vi "OAT Easy Significant Gabor Order Tracking (Digital Tach).vi"(0 "scaled signal [EU]":waveform(dbl)={"t0"=timestamp(0 s since 1904-01-01), "dt"=0.0, "Y"=[]}, 1 "bandwidth":T4={"bandwidth value"=0.5, "bandwidth unit"=enum."Order"} {"bandwidth value" min=0.0 format="%.2f"}, 2 "window info in (auto)":T1={"window type"=10, "window length"=0} {"window type" items=["None"=0, "Hanning"=1, "Hamming"=2, "Blackman-Harris"=3, "Exact Blackman"=4, "Blackman"=5, "Flat Top"=6, "4 Term B-Harris"=7, "7 Term B-Harris"=8, "Low Sidelobe"=9, "Gaussian"=62]; "window length" min=0}, 5 "number of orders (3)":i32=3, 7 "digital tach info":T5={"tacho counts"=[], "counter timebase [Hz]"=20000000.0, "counter task type"=enum."event counting", "counter digit (32)"=32}, 9 "pulse/revolution (1)":i32=1, 11 "error in (no error)":errorcluster, 12 "X axis selection":u16(ring)=2 items=["Time", "Revolution", "RPM"], 13 "phase setting":T2) -> (3 "samples/rev":dbl format="%.2f", 4 "magnitudes (RMS)":cluster{"X":dbl[], "Y":dbl[]}[](array[cluster]) {"Y" format="%.2f"; "X" format="%.2f"}, 6 "phase lags":cluster{"X":dbl[], "Y":dbl[]}[](array[cluster]) {"Y" format="%.2f"; "X" format="%.2f"}, 8 "order waveforms [EU]":waveform(dbl)[](array[waveform]), 10 "unit labels":T3, 14 "orders":dbl[](array[numeric]) format="%.2f", 15 "error out":errorcluster)   [LabVIEW 2017]
doc: "Extracts the most significant orders from <B>scaled signal [EU]</B> and computes <B>magnitudes</B> and <B>phase lags</B> for the significant orders. You can use this polymorphic VI to perform significant order tracking for an analog tachometer signal or a digital tachometer signal. The data type you wire to the <B>analog tach signal</B> input determines the polymorphic instance to use."
uses:
  <vilib>/addons/Sound and Vibration/Order Analysis/Tach Process/SubVIs/digital tach info.ctl
  <vilib>/addons/Sound and Vibration/Order Analysis/Ref Gabor Order Tracking/Mask Bandwidth.ctl
  <vilib>/addons/Sound and Vibration/Order Analysis/Ref Gabor Order Tracking/window information.ctl
  <vilib>/addons/Sound and Vibration/Order Analysis/Tach Process/SubVIs/speed profile.ctl
  <vilib>/addons/Sound and Vibration/Order Analysis/Tach Process/SoundVib_TachProcess.lvlib
  <vilib>/addons/Sound and Vibration/Order Analysis/Gabor Order Tracking/SoundVib_Gabor.lvlib
panel:
  # "OAT Easy Significant Gabor Order Tracking (Digital Tach)"
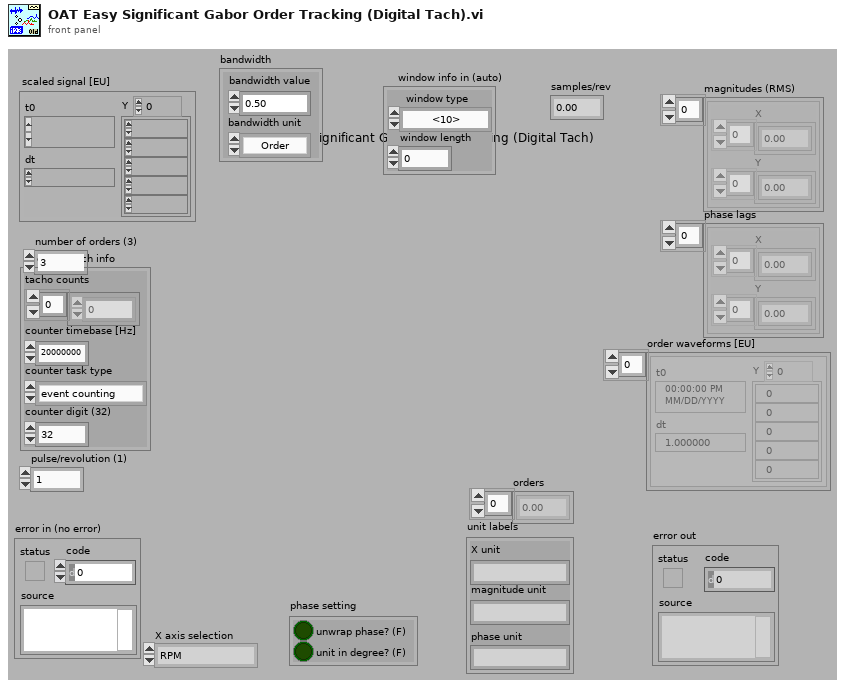
[diagram p1: front panel]
types:
  T1 = typedef "SoundVib_Gabor.lvlib/window information.ctl" = cluster{"window type":u32, "window length":i32}
  T2 = cluster{"unwrap phase? (F)":bool, "unit in degree? (F)":bool}
  T3 = cluster{"X unit":string, "magnitude unit":string, "phase unit":string}
  T4 = typedef "SoundVib_Gabor.lvlib/Mask Bandwidth.ctl" = cluster{"bandwidth value":dbl, "bandwidth unit":enum16{"Order", "Hz"}}
  T5 = typedef "SoundVib_TachProcess.lvlib/digital tach info.ctl" = cluster{"tacho counts":i64[], "counter timebase [Hz]":dbl, "counter task type":enum16{"period measurement", "event counting"}, "counter digit (32)":i32}
  T6 = typedef "SoundVib_TachProcess.lvlib/speed profile.ctl" = cluster{"time [s]":dbl[], "speed [RPM]":dbl[]}
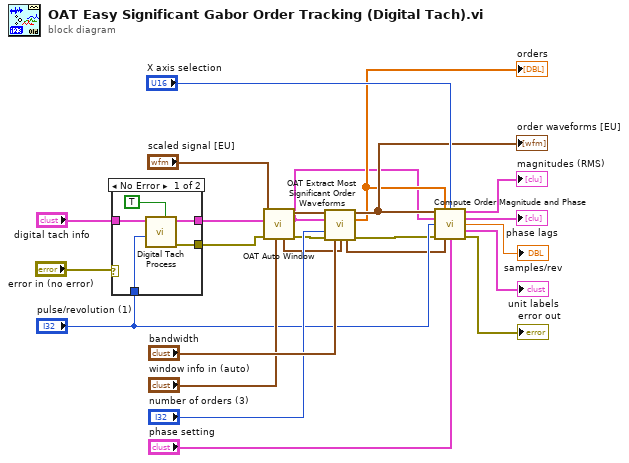
[diagram p0: block diagram]
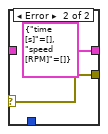
[diagram p2: hidden frame]
diagram:
  n1 = case shown="No Error" "error in (no error)" {
    selector: "error in (no error)" -> [_ w30]
    tunnel: "digital tach info" -> [w29 _]
    tunnel: "pulse/revolution (1)" -> [w28 _]
    tunnel: [w27 T6 {"time [s]"=[], "speed [RPM]"=[]} ("speed profile")] -> w10
    tunnel: [w26 w30] -> w7
    frame No Error {
      n2 = call <vilib>:"Digital Tach Process.vi"("reset? (True)"=TRUE ("reset? (False)"), "pulse/revolution (1)"=w28, "digital tach info"=w29) -> ("error out"=w26:errorcluster, "speed profile"=w27:T6)  [unwired: 6 in, 1 out]
    }
    frame Error {
    }
  }
  n3 = call <vilib>:"OAT Auto Window.vi"("window info in"="window info in (auto)", "error in (no error)"=w7, "speed profile"=w10, "scaled signal [EU]"="scaled signal [EU]") -> ("error out"=w6:errorcluster, "speed profile out"=w3:T6, "scaled signal [EU] out"=w11:waveform(dbl), "window info out"=w9:T1)  [unwired: 4 in]
  n4 = call <vilib>:"OAT Extract Most Significant Order Waveforms.vi"("scaled signal [EU]"=w11, "speed profile"=w3, "number of orders (3)"="number of orders (3)", "error in (no error)"=w6, "bandwidth"="bandwidth", "window info"=w9) -> ("order waveforms [EU]"=w19:waveform(dbl)[], "orders"=w15:dbl[], "actual window info"=w8:T1, "error out"=w5:errorcluster)  [unwired: 5 in, 1 out]
  "orders" <- w15
  "order waveforms [EU]" <- w19
  n5 = call <vilib>:"Compute Order Magnitude and Phase.vi"("order waveforms [EU]"=w19, "orders (1.0)"=w15, "X axis selection"="X axis selection", "speed profile"=w3, "pulse/revolution (1)"="pulse/revolution (1)", "error in (no error)"=w5, "window info"=w8, "phase setting"="phase setting") -> ("magnitudes (RMS)"=→"magnitudes (RMS)":cluster{"X":dbl[], "Y":dbl[]}[], "phase lags"=→"phase lags":cluster{"X":dbl[], "Y":dbl[]}[], "samples/rev"=→"samples/rev":dbl, "unit labels"=→"unit labels":T3, "error out"=→"error out":errorcluster)  [unwired: 3 in]
